vi "Rot A.vi"(8 "error in (no error)":errorcluster) -> (0 "error out":errorcluster, 3 "function return":dbl)   [LabVIEW 2014, in "MASTTCSGET.lvlib"]
doc: "__declspec (dllexport) float RotA();"
uses:
  MASTTCSGET.lvlib
  MASTTCSGET.dll
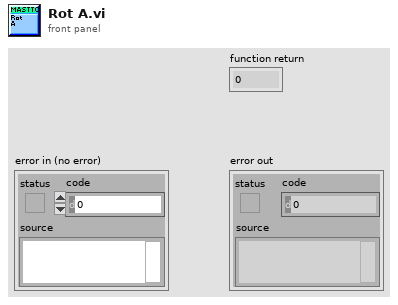
[diagram p1: front panel]
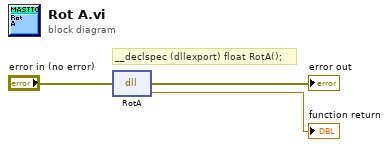
[diagram p0: block diagram]
diagram:
  # "__declspec (dllexport) float RotA();"
  n1 = dll-call lib="C:/Users/sanjay/Desktop/mast_controlsystem/MASTTCSGET.*" fn="RotA"(error in="error in (no error)") -> (error out=→"error out":errorcluster, →"function return":dbl)  [unwired: 2 in, 1 out]
